vi "Remove Col Header Formatting.vi"(8 "error in":errorcluster, 9 "Column Header Strings[] in":string[](array[string]), 11 "MCListbox Refnum in":refnum<vi>) -> (0 "error out":errorcluster, 1 "Column Header Strings[] out":string[](array[string]), 3 "MCListbox Refnum out":refnum<vi>)   [LabVIEW 2012, in "ListBox_XControl.xctl"]
doc: "Remove font markings in column header strings from any previous sorting. Remove bold typeface and directional sort marking from column headers (/\\ or \\/)"
uses:
  ListBox_XControl.xctl
  <vilib>/Utility/miscctls.llb/LVRowAndColumnTypeDef.ctl
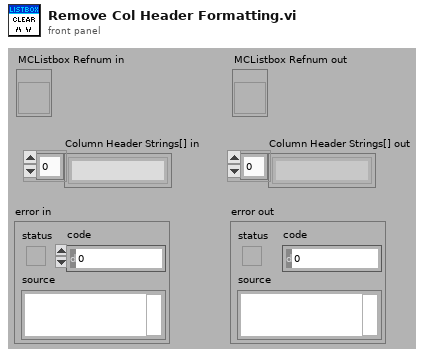
[diagram p1: front panel]
types:
  T1 = typedef "LVRowAndColumnTypeDef.ctl" = cluster{"Row":i32, "Column":i32}
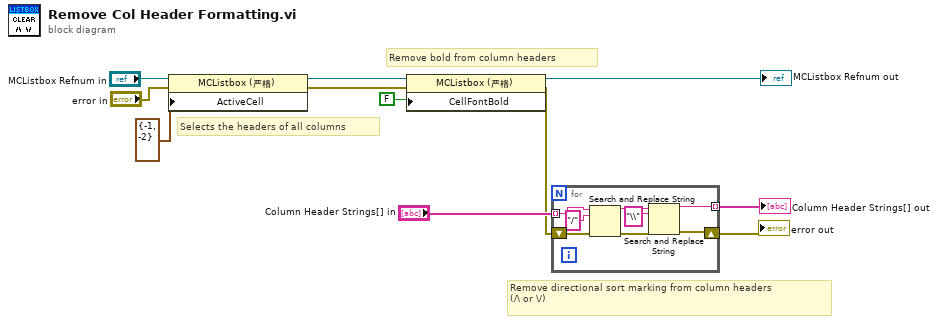
[diagram p0: block diagram]
diagram:
  # "Remove directional sort marking from column headers\n(/\\ or \\/)"
  # "Remove bold from column headers"
  # "Selects the headers of all columns"
  n1 = property on="Property Node" class="MCListbox (严格)"(reference="MCListbox Refnum in", error in="error in", "ActiveCell"=T1 {"Row"=-1, "Column"=-2} ("Active Cell:Active Cell")) -> (reference out=w6:refnum<vi>, error out=w7:errorcluster)
  n2 = property on="Property Node" class="MCListbox (严格)"(reference=w6, error in=w7, "CellFontBold"=FALSE ("Active Cell:Cell Font:Bold")) -> (reference out=→"MCListbox Refnum out":refnum<vi>, error out=w9:errorcluster)
  n3 = for {
    tunnel: "Column Header Strings[] in" -> [w12] mode=indexing
    shift-right: [w14] -> w2
    shift-left: w9 -> [w15]
    tunnel: [w13] -> w1 mode=indexing
    n4 = Search and Replace String(input string=w12, search string="/", error in=w15) -> (result string=w18:string, error out=w17:errorcluster)  [unwired: 5 in, 2 out]
    n5 = Search and Replace String(input string=w18, search string="\\", error in=w17) -> (result string=w13:string, error out=w14:errorcluster)  [unwired: 5 in, 2 out]
  }
  "error out" <- w2
  "Column Header Strings[] out" <- w1
